vi "Configure Device.vi"(8 "error in":errorcluster, 11 "Device in":refnum<class "TE Cooler.lvclass">) -> (0 "error out":errorcluster, 3 "Device out":refnum<class "TE Cooler.lvclass">, 4 "SP":dbl, 5 "Settable?":bool)   [LabVIEW 2015, in "TE Cooler.lvlib" / "TE Cooler.lvclass"]
doc: "This is the configuration method for the Device object. The one parameter that all should have in common and is not dependent on the configuration of the device is the label which is read from the ini file. All devices that use this class should have this in their configuration."
uses:
  TE Cooler.lvclass
  <vilib>/MSR Consulting, LLC/General Reuse/Session APIs/Serial/Serial Session.lvclass
  <vilib>/MSR Consulting, LLC/General Reuse/Session APIs/Session Log/System Log.lvclass
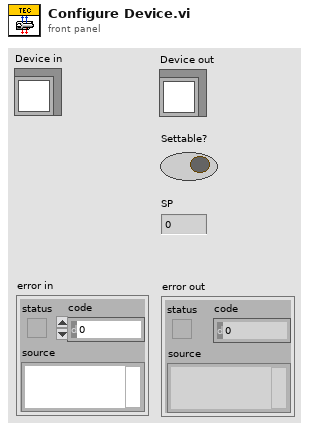
[diagram p1: front panel]
types:
  T1 = typedef "Serial Session.lvclass/Session Handle.ctl" = refnum<data-value>
  T2 = typedef "Config Data.lvclass/Config Session.ctl" = refnum<data-value>
  T3 = typedef "Session - Root.lvclass/Session Handle.ctl" = refnum<data-value>
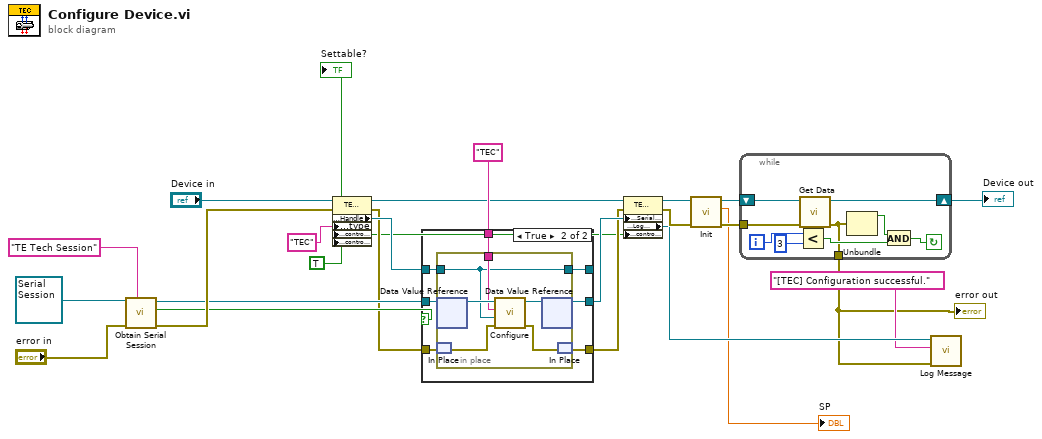
[diagram p0: block diagram]
diagram:
  w3 = TRUE ("controller_")
  n1 = call <vilib>:"Obtain Serial Session.vi"("Session Name ()"="TE Tech Session", "error in"="error in", "Serial Session in"=refnum<class "Serial Session.lvclass"> refnum) -> ("error out"=w21:errorcluster, "created new?"=w18:bool, "hSerial"=w17:T1)  [unwired: 6 in]
  n2 = property class="TE Tech"(reference="Device in", error in=w21, "Accessors:type"="TEC" ("type"), "Accessors:controller_"=w3, "Accessors:controller_"=w3) -> (reference out=w16:refnum<class "TE Cooler.lvclass">, error out=w8:errorcluster, "Accessors:Handle"=w19:T2)
  n3 = case shown="True" w18 {
    tunnel: w17 -> [w27 w34]
    tunnel: w8 -> [w26 w30]
    tunnel: [w27 w33] -> w15
    tunnel: [w26 w32] -> w7
    tunnel: w19 -> [w25 w31]
    tunnel: [w25 w29] -> _
    tunnel: "TEC" ("section") -> [_ w28]
    frame False {
    }
    frame True {
      n4 = in-place {
        in-place-border: w31 -> [w35]
        in-place-border: w28 -> [w36]
        in-place-border: [w35] -> w29
        n5 = in-place-dvr #1(w34) -> (w40:refnum<class "Serial Session.lvclass">)  [unwired: 1 out]
        n6 = in-place-match #2(w30) -> (w39:errorcluster)
        n7 = call <vilib>:"Configure.vi"("error in"=w39, "Config Handle"=w35, "section"=w36, "Serial Session in"=w40) -> ("error out"=w38:errorcluster, "Serial Session out"=w37:refnum<class "Serial Session.lvclass">)  [unwired: 6 in]
        n8 = in-place-dvr #1(w37) -> (w33:T1)  [unwired: 1 out]
        n9 = in-place-match #2(w38) -> (w32:errorcluster)
      }
    }
  }
  n10 = property class="TE Tech"(reference=w16, error in=w7, "Accessors:Serial Session"=w15, "Accessors:controller_"=w3) -> (reference out=w14:refnum<class "TE Cooler.lvclass">, error out=w13:errorcluster, "Accessors:Log Session"=w10:T3)
  n11 = call-dynamic "Init.vi"("error in"=w13, "TE Cooler in"=w14) -> ("error out"=w11:errorcluster, "SP"=→"SP":dbl, "TE Cooler out"=w12:refnum<class "TE Cooler.lvclass">)  [unwired: 7 in]
  n12 = while {
    shift-right: [w48] -> w5
    shift-left: w12 -> [w49]
    tunnel: [w42] -> w6
    tunnel: w11 -> [w41]
    i -> [w45]
    stop <- w46 continue-if-true
    n13 = Less?(x=w45, y=3) -> (x < y?=w43:bool)
    n14 = call-dynamic "Get Data.vi"("error in"=w41, "TE Cooler in"=w49) -> ("error out"=w42:errorcluster, "TE Cooler out"=w48:refnum<class "TE Cooler.lvclass">)  [unwired: 7 in, 1 out]
    n15 = Unbundle(w42) -> ("status"=w47:bool)  [unwired: 2 out]
    n16 = And(x=w47, y=w43) -> (x .and. y?=w46:bool)
  }
  "error out" <- w6
  "Device out" <- w5
  n17 = call <vilib>:"Log Message.vi"("error in"=w6, "MSG In"="[TEC] Configuration successful.", "session in"=w10) -> ()  [unwired: 7 in, 2 out]
  "Settable?" <- w3
